vi "Read All Keys.vi"(8 "error in":errorcluster, 11 "E2E configuration in":refnum<class "E2E Tag Exchange configuration.lvclass">) -> (0 "error out":errorcluster, 1 "Values":string[](array[string]), 2 "Keys":string[](array[string]), 3 "E2E configuration out":refnum<class "E2E Tag Exchange configuration.lvclass">)   [LabVIEW 2015, in "E2E Tag Exchange configuration.lvclass"]
uses:
  E2E Tag Exchange configuration.lvclass
  E2E Tag Exchange configuration.lvclass/E2E Tag Exchange configuration.ctl
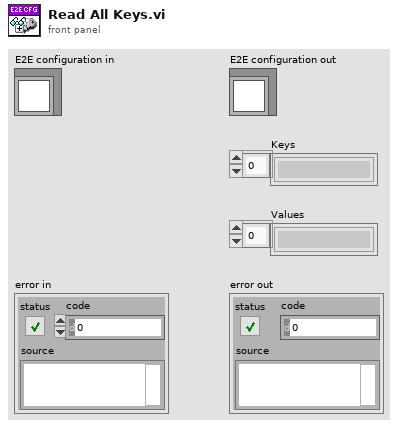
[diagram p1: front panel]
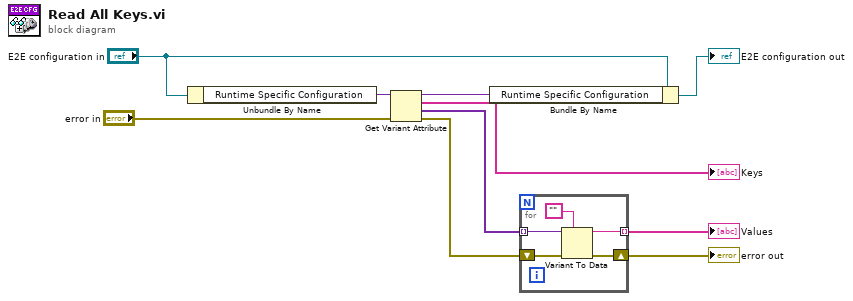
[diagram p0: block diagram]
diagram:
  n1 = Unbundle By Name("E2E configuration in") -> ("Runtime Specific Configuration"=w10:variant)
  n2 = Get Variant Attribute(Variant=w10, error in="error in") -> (duplicate Variant=w8:variant, names=→"Keys":string[], values=w4:variant[], error out=w2:errorcluster)  [unwired: 2 in]
  n3 = Bundle By Name(cluster="E2E configuration in", "Runtime Specific Configuration"=w8) -> (→"E2E configuration out":refnum<class "E2E Tag Exchange configuration.lvclass">)
  n4 = for {
    tunnel: w4 -> [w15] mode=indexing
    tunnel: [w13] -> w3 mode=indexing
    shift-right: [w11] -> w1
    shift-left: w2 -> [w12]
    n5 = Variant To Data(error in=w12, type="", Variant=w15) -> (data=w13:string, error out=w11:errorcluster)
  }
  "error out" <- w1
  "Values" <- w3
